vi "Get Component Settings.vi"(8 "error in (no error)":errorcluster, 11 "Item Ref in":T2 format="%.0x") -> (0 "error out":errorcluster, 2 "component settings":T1[](array[typedef]), 3 "Item Ref out":T2 format="%.0x")   [LabVIEW 2019, in "DSF Shared.lvlib"]
uses:
  DSF Shared.lvlib
  <vilib>/NI VeriStand/Custom Device API/Custom Device API.lvlib
  DSF Core.lvlibp/Typedefs/DSF Settings Info.ctl
  <vilib>/NI VeriStand/Custom Device API/Get Item Property (Variant).vi
  <vilib>/NI VeriStand/Custom Device API/Custom Device Item Ref.ctl
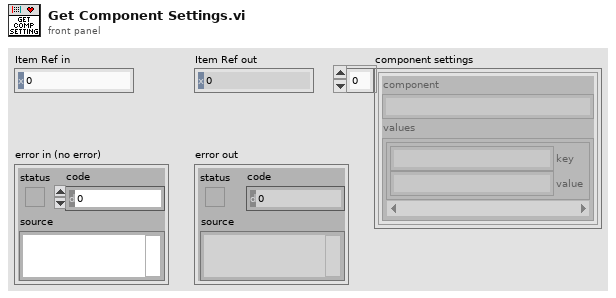
[diagram p1: front panel]
types:
  T1 = typedef "DSF Core.lvlibp/DSF Settings Info.ctl" = cluster{"component":string, "values":cluster{"key":string, "value":string}[]}
  T2 = typedef "Custom Device API.lvlib/Custom Device Item Ref.ctl" = u64
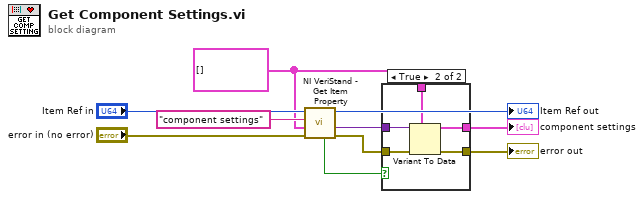
[diagram p0: block diagram]
diagram:
  w1 = T1[] [] ("component settings")
  n1 = call-poly <vilib>:"NI VeriStand - Get Item Property.vi"("error in (no error)"="error in (no error)", "Default Value"=w1, "Property Name"="component settings" ("dsf options"), "Item Ref in"="Item Ref in") -> ("error out"=w8:errorcluster, "Value"=w7:variant, "Item Ref out"=→"Item Ref out":T2, "Found?"=w4:bool)  [unwired: 4 in]
  n2 = case shown="True" w4 {
    tunnel: w8 -> [w11 w17]
    tunnel: w1 -> [w12 w16]
    tunnel: w7 -> [_ w15]
    tunnel: [w11 w14] -> w6
    tunnel: [w12 w13] -> w2
    frame False {
    }
    frame True {
      n3 = Variant To Data(error in=w17, type=w16, Variant=w15) -> (data=w13:T1[], error out=w14:errorcluster)
    }
  }
  "error out" <- w6
  "component settings" <- w2
